vi "Randomize.vi"() -> (1 "Theta":dbl, 2 "Beta":dbl, 3 "Alpha":dbl)   [LabVIEW 2019]
uses:
  <vilib>/numeric/Random Number (Range) U64.vi
  <vilib>/numeric/sub_Random U32.vi
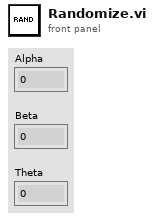
[diagram p1: front panel]
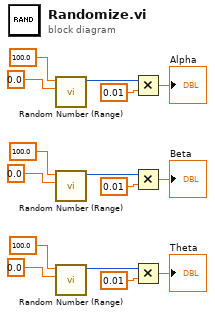
[diagram p0: block diagram]
diagram:
  n1 = call-poly <vilib>:"Random Number (Range).vi"("lower bound (0)"=0.0, "upper bound (100)"=100.0) -> ("number"=w3:u64)  [unwired: 9 in]
  n2 = call-poly <vilib>:"Random Number (Range).vi"("lower bound (0)"=0.0, "upper bound (100)"=100.0) -> ("number"=w7:u64)  [unwired: 9 in]
  n3 = call-poly <vilib>:"Random Number (Range).vi"("lower bound (0)"=0.0, "upper bound (100)"=100.0) -> ("number"=w11:u64)  [unwired: 9 in]
  n4 = Multiply(x=w3, y=0.01) -> (x*y=→"Alpha":dbl)
  n5 = Multiply(x=w7, y=0.01) -> (x*y=→"Beta":dbl)
  n6 = Multiply(x=w11, y=0.01) -> (x*y=→"Theta":dbl)
